vi "Is Cluster.vi"(8 "Error In":errorcluster) -> (0 "Error Out":errorcluster)   [LabVIEW 2018, in "Tests.lvlib" / "Toolkit.lvlib"]
uses:
  Toolkit.lvlib
  <vilib>/Utility/traverseref.llb/TRef TravTarget.ctl
  <vilib>/addons/_JKI Toolkits/Caraya/classes/Test/Test.lvclass
  <vilib>/addons/_JKI Toolkits/Caraya/classes/Assert/Assert.lvclass
  <vilib>/Utility/traverseref.llb/VI Scripting - Traverse.lvlib
  src/Toolkit/Toolkit.lvlib
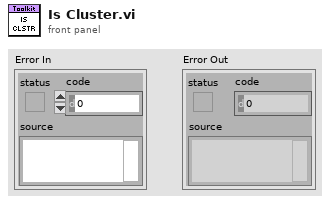
[diagram p1: front panel]
types:
  T1 = typedef "TRef TravTarget.ctl" = enum16{"FP", "BD", "Other"}
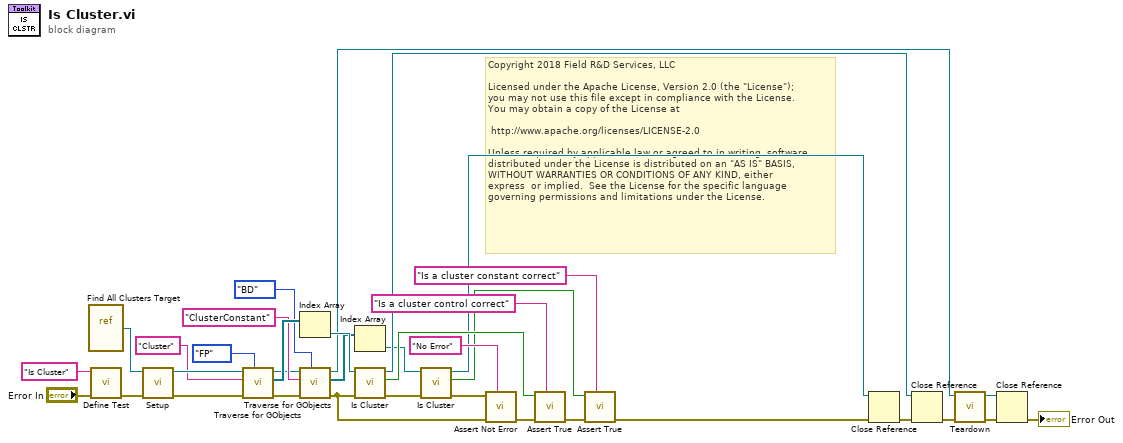
[diagram p0: block diagram]
diagram:
  # "Copyright 2018 Field R&D Services, LLC\n\nLicensed under the Apache License, Version 2.0 (the \"License\");\nyou may not use this file except in compliance with the License.\nYou may obtain a copy of the License at\n\n\thttp://www.apache.org/licenses/LICENSE-2.0\n\nUnless required by applicable law or agreed to in writing, software\ndistributed under the License is distributed on an \"AS IS\" BASIS,\nWITHOUT WARRANTIES OR CONDITIONS OF ANY KIND, either \nexpress  or implied.  See the License for the specific language \ngoverning permissions and limitations under the License."
  n1 = vi-ref "Find All Clusters Target.vi"() -> (w32:refnum<vi>)
  n2 = call <vilib>:"Define Test.vi"("error in (no error)"="Error In", "Label (VI Title)"="Is Cluster") -> ("error out"=w33:errorcluster)  [unwired: 9 in]
  n3 = call "Setup.vi"("Error In"=w33, "VI In"=w32) -> ("Error Out"=w16:errorcluster, "VI Out"=w23:refnum<vi>)  [unwired: 8 in]
  n4 = call <vilib>:"Traverse for GObjects.vi"("Traverse Target"=TRef_TravTarget."FP", "error in (no error)"=w16, "Class Name"="Cluster", "VI Refnum"=w23) -> ("error out"=w15:errorcluster, "References"=w20:refnum<vi>[], "dup VI Refnum"=w12:refnum<vi>)  [unwired: 4 in, 1 out]
  n5 = Index Array(array=w20) -> (element=w19:refnum<vi>)  [unwired: 1 in]
  n6 = call <vilib>:"Traverse for GObjects.vi"("Traverse Target"=TRef_TravTarget."BD", "error in (no error)"=w15, "Class Name"="ClusterConstant", "VI Refnum"=w12) -> ("error out"=w10:errorcluster, "References"=w9:refnum<vi>[], "dup VI Refnum"=w11:refnum<vi>)  [unwired: 4 in, 1 out]
  n7 = Index Array(array=w9) -> (element=w8:refnum<vi>)  [unwired: 1 in]
  n8 = call "Is Cluster.vi"("Error In"=w10, "GObject In"=w19) -> ("Error Out"=w7:errorcluster, "Cluster?"=w17:bool, "GObject Out"=w18:refnum<vi>)  [unwired: 7 in]
  n9 = call "Is Cluster.vi"("Error In"=w7, "GObject In"=w8) -> ("Error Out"=w6:errorcluster, "Cluster?"=w5:bool, "GObject Out"=w2:refnum<vi>)  [unwired: 7 in]
  n10 = call <vilib>:"Assert Not Error.vi"("Label"="No Error", "error in (no error)"=w10, "Not Error?"=w6) -> ("error out"=w25:errorcluster)  [unwired: 8 in]
  n11 = call <vilib>:"Assert True.vi"("Label"="Is a cluster control correct", "error in (no error)"=w25, "True?"=w17) -> ("error out"=w29:errorcluster)  [unwired: 8 in]
  n12 = call <vilib>:"Assert True.vi"("Label"="Is a cluster constant correct", "error in (no error)"=w29, "True?"=w5) -> ("error out"=w4:errorcluster)  [unwired: 8 in]
  n13 = Close Reference(reference=w2, error in (no error)=w4) -> (error out=w3:errorcluster)
  n14 = Close Reference(reference=w18, error in (no error)=w3) -> (error out=w24:errorcluster)
  n15 = call "Teardown.vi"("Error In"=w24, "VI In"=w11) -> ("Error Out"=w27:errorcluster, "VI Out"=w28:refnum<vi>)  [unwired: 8 in]
  n16 = Close Reference(reference=w28, error in (no error)=w27) -> (error out=→"Error Out":errorcluster)
